vi "Panel induced velocity at point P.vi"(1 "P":sgl[](array[numeric]), 2 "Triangle panel":T1={"V0"=[], "V1"=[], "V2"=[], "E0"=[], "E1"=[], "E2"=[], "n^"=[], "Pc"=[], "Gamma'"=0.0, "V_transp."=0.0, "E0 link"=-1, "E1 link"=-1, "E2 link"=-1}) -> (0 "U / G'":sgl[](array[numeric]))   [LabVIEW 2017]
uses:
  ctls/Triangle panel.ctl
panel:
  # "PN 22/10/17"
  # "Vertices"
  # "Edges"
  # "Unit normal"
  # "Control point"
  # "Edge\nlinks \n(tri index)"
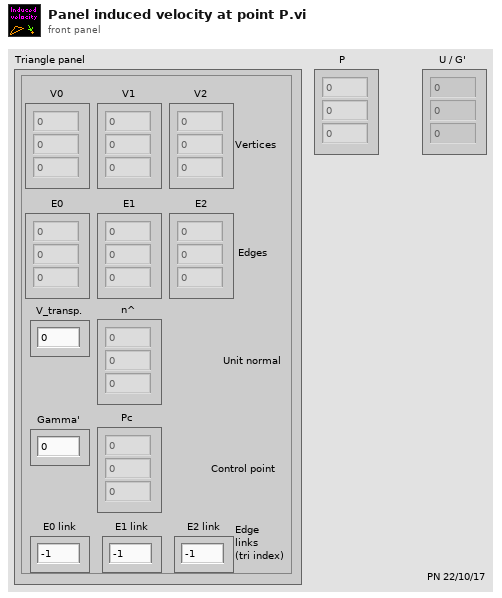
[diagram p1: front panel]
types:
  T1 = typedef "Triangle panel.ctl" = cluster{"V0":sgl[], "V1":sgl[], "V2":sgl[], "E0":sgl[], "E1":sgl[], "E2":sgl[], "n^":sgl[], "Pc":sgl[], "Gamma'":sgl, "V_transp.":sgl, "E0 link":i32, "E1 link":i32, "E2 link":i32}
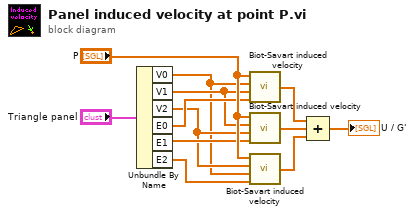
[diagram p0: block diagram]
diagram:
  n1 = Unbundle By Name("Triangle panel") -> ("V0"=w6:sgl[], "V1"=w9:sgl[], "V2"=w7:sgl[], "E0"=w10:sgl[], "E1"=w8:sgl[], "E2"=w5:sgl[])
  n2 = call "Biot-Savart induced velocity.vi"("E"=w10, "P1"=w9, "P0"=w6, "P"="P") -> ("U / G'"=w4:sgl[])
  n3 = call "Biot-Savart induced velocity.vi"("E"=w8, "P1"=w7, "P0"=w9, "P"="P") -> ("U / G'"=w3:sgl[])
  n4 = call "Biot-Savart induced velocity.vi"("E"=w5, "P1"=w6, "P0"=w7, "P"="P") -> ("U / G'"=w2:sgl[])
  n5 = Compound Arithmetic op=ADD(w4, w3, w2) -> (→"U / G'":sgl[])
